vi "Add Default Free.vi"(8 "error in (no error)":errorcluster, 10 "ToModBus":bool, 11 "Strain in":refnum<class "Strain.lvclass">) -> (0 "error out":errorcluster, 3 "Strain out":refnum<class "Strain.lvclass">)   [LabVIEW 2018, in "Measurement Channels.lvlib" / "Strain.lvclass"]
uses:
  Strain.lvclass
  Strain.lvclass/Strain.ctl
  Class Channel/Channel.lvclass
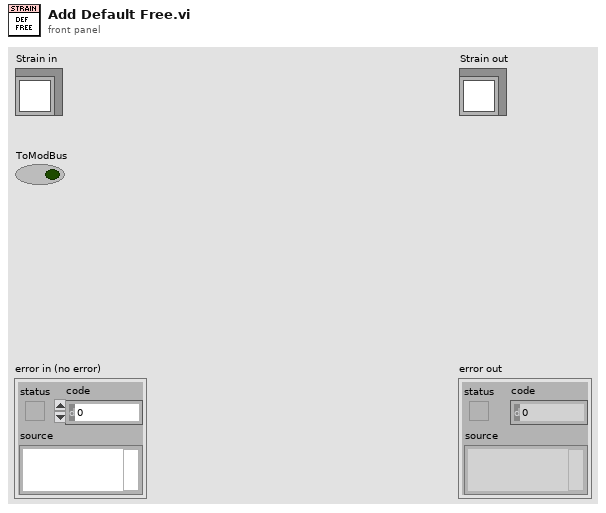
[diagram p1: front panel]
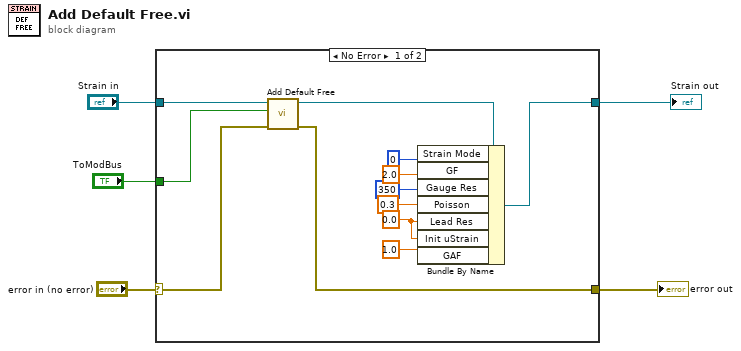
[diagram p0: block diagram]
diagram:
  n1 = case shown="No Error" "error in (no error)" {
    selector: "error in (no error)" -> [w7 w18]
    tunnel: "Strain in" -> [w17 w19]
    tunnel: "ToModBus" -> [w16 _]
    tunnel: [w14 w19] -> w3
    tunnel: [w13 w18] -> w2
    frame No Error {
      w9 = 0.0 ("Lead Res")
      n2 = call-parent "Add Default Free.vi"("error in (no error)"=w7, "ToModBus"=w16, "Channel in"=w17) -> ("error out"=w13:errorcluster, "Channel out"=w15:refnum<class "Strain.lvclass">)  [unwired: 7 in]
      n3 = Bundle By Name(cluster=w15, "Strain Mode"=u16 0, "GF"=2.0, "Gauge Res"=350, "Poisson"=0.3, "Lead Res"=w9, "Init uStrain"=w9, "GAF"=1.0) -> (w14:refnum<class "Strain.lvclass">)
    }
    frame Error {
    }
  }
  "error out" <- w2
  "Strain out" <- w3
